vi "Store.vi"(8 "error in (no error)":errorcluster, 11 "PredictiveMaintenance in":refnum<class "PredictiveMaintenance.lvclass">) -> (0 "error out":errorcluster, 3 "PredictiveMaintenance out":refnum<class "PredictiveMaintenance.lvclass">)   [LabVIEW 2019, in "PredictiveMaintenance.lvlib" / "PredictiveMaintenance.lvclass"]
uses:
  PredictiveMaintenance.lvclass
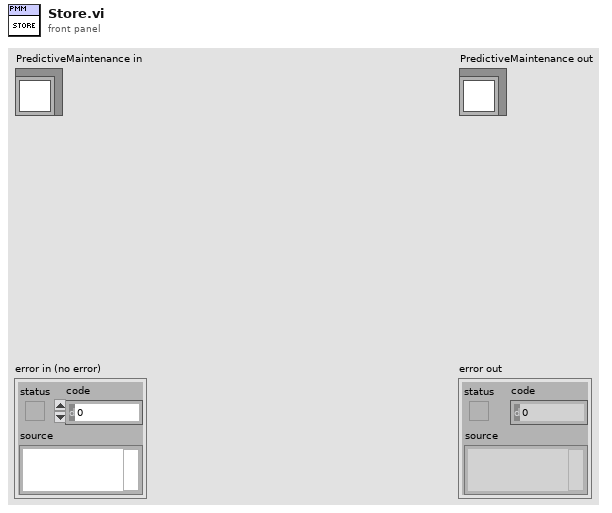
[diagram p1: front panel]
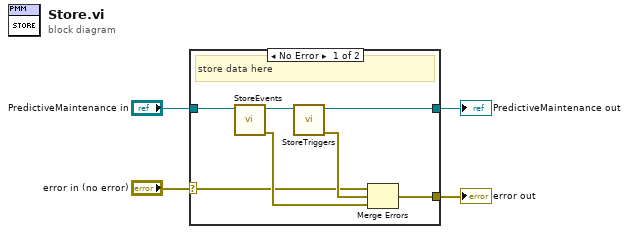
[diagram p0: block diagram]
diagram:
  n1 = case shown="No Error" "error in (no error)" {
    selector: "error in (no error)" -> [w5 w13]
    tunnel: [w9 w13] -> w3
    tunnel: [w10 w12] -> w1
    tunnel: "PredictiveMaintenance in" -> [w6 w12]
    frame No Error {
      # "store data here"
      n2 = call "StoreEvents.vi"("PredictiveMaintenance.lvlib:PredictiveMaintenance_IN"=w6) -> ("error out"=w7:errorcluster, "PredictiveMaintenance.lvlib:PredictiveMaintenance_OUT"=w11:refnum<class "PredictiveMaintenance.lvclass">)  [unwired: 9 in]
      n3 = call "StoreTriggers.vi"("PredictiveMaintenance.lvlib:PredictiveMaintenance_IN"=w11) -> ("error out"=w8:errorcluster, "PredictiveMaintenance.lvlib:PredictiveMaintenance_OUT"=w10:refnum<class "PredictiveMaintenance.lvclass">)  [unwired: 9 in]
      n4 = Merge Errors(w5, w8, w7) -> (w9:errorcluster)
    }
    frame Error {
    }
  }
  "error out" <- w3
  "PredictiveMaintenance out" <- w1
